vi "产生多组数值.vi"() -> (0 "牌3":dbl, 1 "牌4":dbl, 2 "牌2":dbl, 3 "牌1":dbl, 4 "牌4值":dbl, 5 "牌3值":dbl, 6 "牌2值":dbl, 7 "牌1值":dbl)   [LabVIEW 2014]
uses:
  <vilib>/Utility/file.llb/Write To Spreadsheet File (DBL).vi
panel:
  in  "数值":i32
  out "大小":i32[](array[numeric])
  out "添加的数组":dbl[][](array[numeric])
  out "布尔":bool
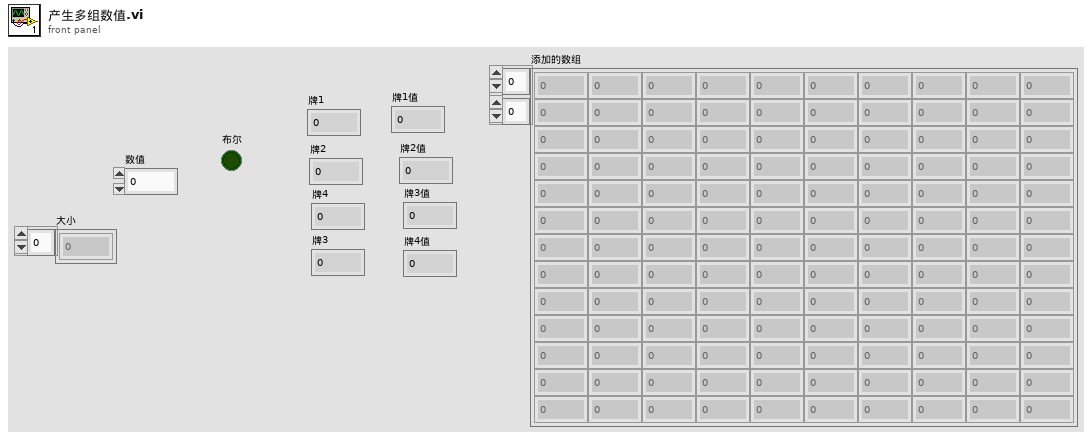
[diagram p1: front panel]
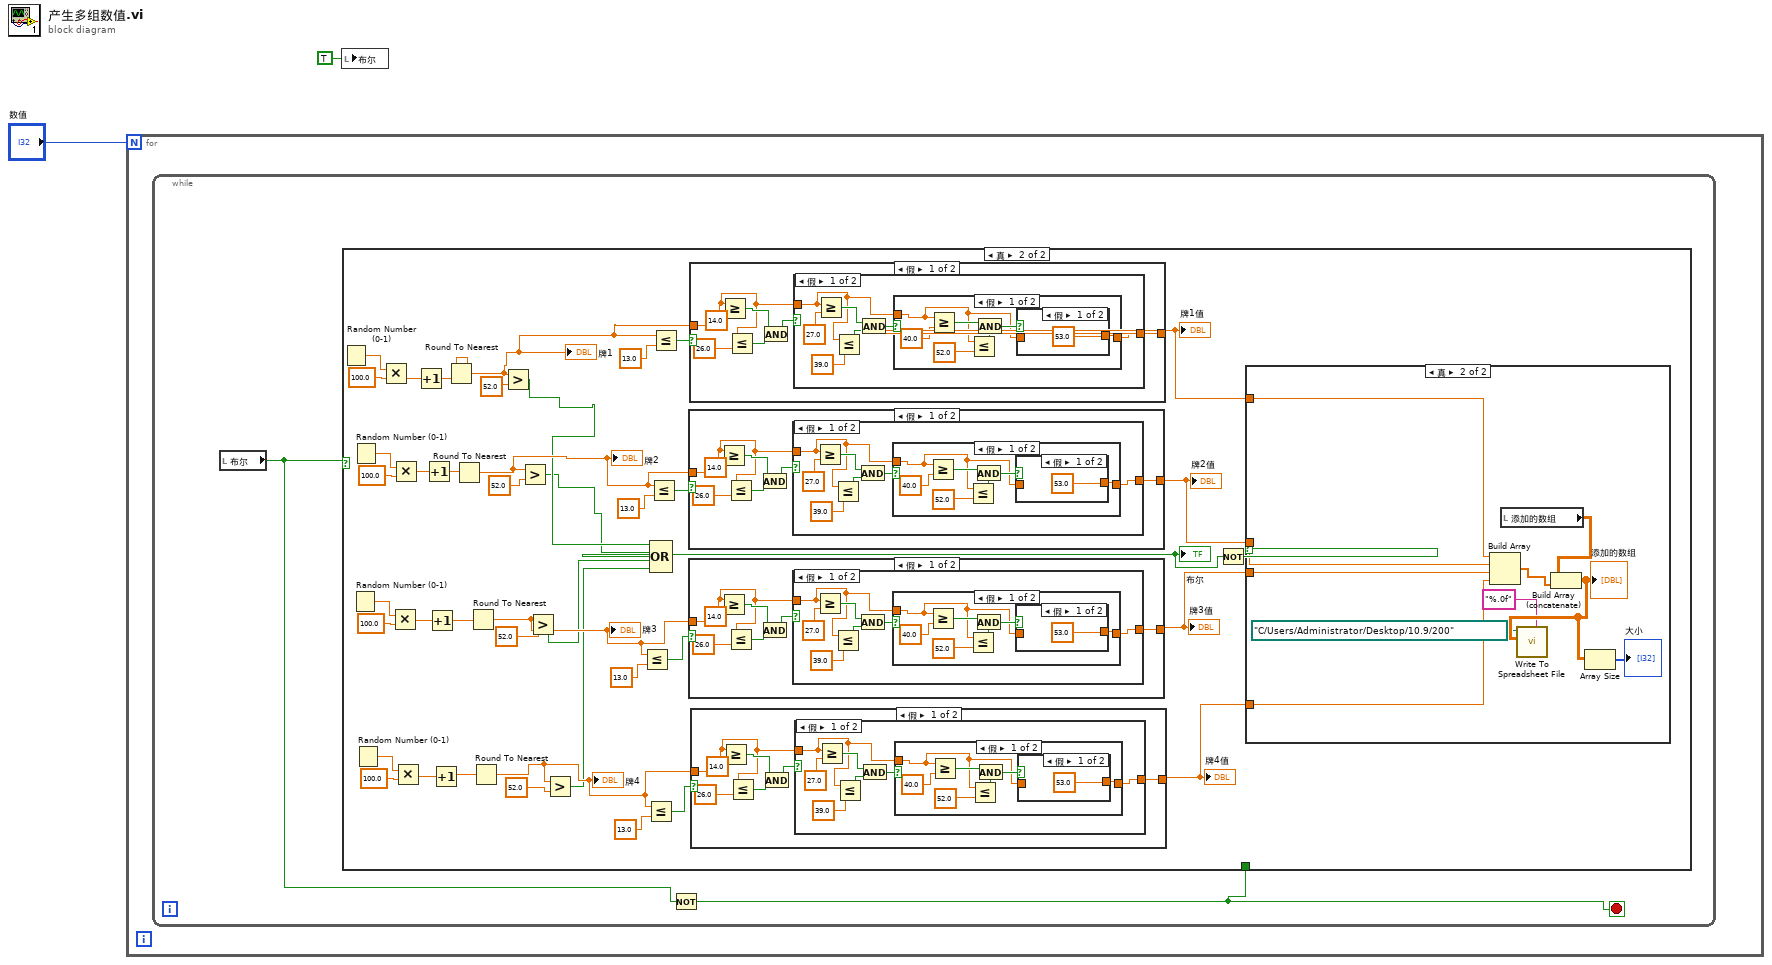
[diagram p0: block diagram]
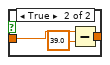
[diagram p4: hidden frame]
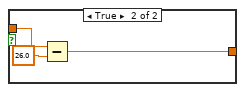
[diagram p5: hidden frame]
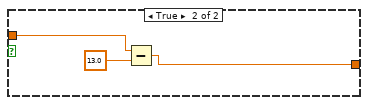
[diagram p6: hidden frame]
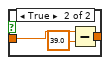
[diagram p8: hidden frame]
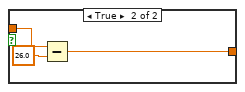
[diagram p9: hidden frame]
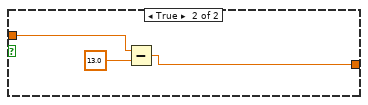
[diagram p10: hidden frame]
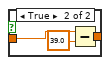
[diagram p12: hidden frame]
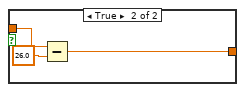
[diagram p13: hidden frame]
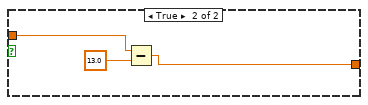
[diagram p14: hidden frame]
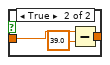
[diagram p16: hidden frame]
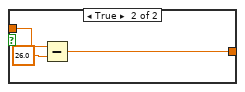
[diagram p17: hidden frame]
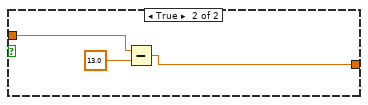
[diagram p18: hidden frame]
diagram:
  n1 = for {
    N: "数值" -> [_]
    n2 = while {
      stop <- w3 stop-if-true
      n3 = local read "布尔"() -> (w4:bool)
      n4 = Not(x=w4) -> (.not. x?=w3:bool)
      n5 = case shown="真" w4 {
        tunnel: w3 -> [_ _]
        frame False {
        }
        frame True {
          n6 = Random Number (0-1)() -> (number: 0 to 1=w39:dbl)
          n7 = Random Number (0-1)() -> (number: 0 to 1=w42:dbl)
          n8 = Random Number (0-1)() -> (number: 0 to 1=w46:dbl)
          n9 = Random Number (0-1)() -> (number: 0 to 1=w43:dbl)
          n10 = Multiply(x=w39, y=100.0) -> (x*y=w22:dbl)
          n11 = Multiply(x=w42, y=100.0) -> (x*y=w13:dbl)
          n12 = Multiply(x=w46, y=100.0) -> (x*y=w11:dbl)
          n13 = Multiply(x=w43, y=100.0) -> (x*y=w15:dbl)
          n14 = Increment(x=w22) -> (x+1=w21:dbl)
          n15 = Increment(x=w11) -> (x+1=w12:dbl)
          n16 = Increment(x=w13) -> (x+1=w14:dbl)
          n17 = Increment(x=w15) -> (x+1=w16:dbl)
          n18 = Round To Nearest(number=w21) -> (nearest integer value=w27:dbl)
          "牌1" <- w27
          n19 = Round To Nearest(number=w12) -> (nearest integer value=w28:dbl)
          "牌2" <- w28
          n20 = Round To Nearest(number=w14) -> (nearest integer value=w29:dbl)
          "牌3" <- w29
          n21 = Round To Nearest(number=w16) -> (nearest integer value=w30:dbl)
          "牌4" <- w30
          n22 = Greater?(x=w27, y=52.0) -> (0:w20:bool)
          n23 = Greater?(x=w28, y=52.0) -> (0:w19:bool)
          n24 = Greater?(x=w29, y=52.0) -> (0:w18:bool)
          n25 = Greater?(x=w30, y=52.0) -> (0:w17:bool)
          n26 = Less Or Equal?(x=w29, y=13.0) -> (x <= y?=w24:bool)
          n27 = Less Or Equal?(x=w30, y=13.0) -> (x <= y?=w23:bool)
          n28 = Less Or Equal?(x=w28, y=13.0) -> (x <= y?=w25:bool)
          n29 = Compound Arithmetic op=OR(w20, w19, w18, w17) -> (w6:bool)
          "布尔" <- w6
          n30 = Less Or Equal?(x=w27, y=13.0) -> (x <= y?=w26:bool)
          n31 = case shown="假" w25 {
            tunnel: [w121 w152] -> w9
            tunnel: w28 -> [w122 w152]
            frame False {
              n32 = Greater Or Equal?(x=w122, y=14.0) -> (x >= y?=w124:bool)
              n33 = Less Or Equal?(x=w122, y=26.0) -> (x <= y?=w125:bool)
              n34 = And(x=w124, y=w125) -> (x .and. y?=w123:bool)
              n35 = case shown="假" w123 {
                tunnel: w122 -> [w129 w150]
                tunnel: [w128 w149] -> w121
                frame False {
                  n36 = Greater Or Equal?(x=w129, y=27.0) -> (x >= y?=w132:bool)
                  n37 = Less Or Equal?(x=w129, y=39.0) -> (x <= y?=w131:bool)
                  n38 = And(x=w132, y=w131) -> (x .and. y?=w130:bool)
                  n39 = case shown="假" w130 {
                    tunnel: w129 -> [w137 w148]
                    tunnel: [w136 w146] -> w128
                    frame False {
                      n40 = Greater Or Equal?(x=w137, y=40.0) -> (x >= y?=w139:bool)
                      n41 = Less Or Equal?(x=w137, y=52.0) -> (x <= y?=w135:bool)
                      n42 = And(x=w139, y=w135) -> (x .and. y?=w138:bool)
                      n43 = case shown="假" w138 {
                        tunnel: w137 -> [_ w144]
                        tunnel: [53.0 ("y") w143] -> w136
                        frame False {
                        }
                        frame True {
                          n44 = Subtract(x=w144, y=39.0) -> (x-y=w143:dbl)
                        }
                      }
                    }
                    frame True {
                      n45 = Subtract(x=w148, y=26.0) -> (x-y=w146:dbl)
                    }
                  }
                }
                frame True {
                  n46 = Subtract(x=w150, y=13.0) -> (x-y=w149:dbl)
                }
              }
            }
            frame True {
            }
          }
          "牌2值" <- w9
          n47 = case shown="假" w24 {
            tunnel: [w89 w120] -> w8
            tunnel: w29 -> [w90 w120]
            frame False {
              n48 = Greater Or Equal?(x=w90, y=14.0) -> (x >= y?=w92:bool)
              n49 = Less Or Equal?(x=w90, y=26.0) -> (x <= y?=w93:bool)
              n50 = And(x=w92, y=w93) -> (x .and. y?=w91:bool)
              n51 = case shown="假" w91 {
                tunnel: w90 -> [w97 w118]
                tunnel: [w96 w117] -> w89
                frame False {
                  n52 = Greater Or Equal?(x=w97, y=27.0) -> (x >= y?=w100:bool)
                  n53 = Less Or Equal?(x=w97, y=39.0) -> (x <= y?=w99:bool)
                  n54 = And(x=w100, y=w99) -> (x .and. y?=w98:bool)
                  n55 = case shown="假" w98 {
                    tunnel: w97 -> [w105 w116]
                    tunnel: [w104 w114] -> w96
                    frame False {
                      n56 = Greater Or Equal?(x=w105, y=40.0) -> (x >= y?=w107:bool)
                      n57 = Less Or Equal?(x=w105, y=52.0) -> (x <= y?=w103:bool)
                      n58 = And(x=w107, y=w103) -> (x .and. y?=w106:bool)
                      n59 = case shown="假" w106 {
                        tunnel: w105 -> [_ w112]
                        tunnel: [53.0 ("y") w111] -> w104
                        frame False {
                        }
                        frame True {
                          n60 = Subtract(x=w112, y=39.0) -> (x-y=w111:dbl)
                        }
                      }
                    }
                    frame True {
                      n61 = Subtract(x=w116, y=26.0) -> (x-y=w114:dbl)
                    }
                  }
                }
                frame True {
                  n62 = Subtract(x=w118, y=13.0) -> (x-y=w117:dbl)
                }
              }
            }
            frame True {
            }
          }
          "牌3值" <- w8
          n63 = case shown="假" w26 {
            tunnel: [w153 w184] -> w10
            tunnel: w27 -> [w154 w184]
            frame False {
              n64 = Greater Or Equal?(x=w154, y=14.0) -> (x >= y?=w156:bool)
              n65 = Less Or Equal?(x=w154, y=26.0) -> (x <= y?=w157:bool)
              n66 = And(x=w156, y=w157) -> (x .and. y?=w155:bool)
              n67 = case shown="假" w155 {
                tunnel: w154 -> [w161 w182]
                tunnel: [w160 w181] -> w153
                frame False {
                  n68 = Greater Or Equal?(x=w161, y=27.0) -> (x >= y?=w164:bool)
                  n69 = Less Or Equal?(x=w161, y=39.0) -> (x <= y?=w163:bool)
                  n70 = And(x=w164, y=w163) -> (x .and. y?=w162:bool)
                  n71 = case shown="假" w162 {
                    tunnel: w161 -> [w169 w180]
                    tunnel: [w168 w178] -> w160
                    frame False {
                      n72 = Greater Or Equal?(x=w169, y=40.0) -> (x >= y?=w171:bool)
                      n73 = Less Or Equal?(x=w169, y=52.0) -> (x <= y?=w167:bool)
                      n74 = And(x=w171, y=w167) -> (x .and. y?=w170:bool)
                      n75 = case shown="假" w170 {
                        tunnel: w169 -> [_ w176]
                        tunnel: [53.0 ("y") w175] -> w168
                        frame False {
                        }
                        frame True {
                          n76 = Subtract(x=w176, y=39.0) -> (x-y=w175:dbl)
                        }
                      }
                    }
                    frame True {
                      n77 = Subtract(x=w180, y=26.0) -> (x-y=w178:dbl)
                    }
                  }
                }
                frame True {
                  n78 = Subtract(x=w182, y=13.0) -> (x-y=w181:dbl)
                }
              }
            }
            frame True {
            }
          }
          "牌1值" <- w10
          n79 = case shown="假" w23 {
            tunnel: [w57 w88] -> w7
            tunnel: w30 -> [w58 w88]
            frame False {
              n80 = Greater Or Equal?(x=w58, y=14.0) -> (x >= y?=w60:bool)
              n81 = Less Or Equal?(x=w58, y=26.0) -> (x <= y?=w61:bool)
              n82 = And(x=w60, y=w61) -> (x .and. y?=w59:bool)
              n83 = case shown="假" w59 {
                tunnel: w58 -> [w65 w86]
                tunnel: [w64 w85] -> w57
                frame False {
                  n84 = Greater Or Equal?(x=w65, y=27.0) -> (x >= y?=w68:bool)
                  n85 = Less Or Equal?(x=w65, y=39.0) -> (x <= y?=w67:bool)
                  n86 = And(x=w68, y=w67) -> (x .and. y?=w66:bool)
                  n87 = case shown="假" w66 {
                    tunnel: w65 -> [w73 w84]
                    tunnel: [w72 w82] -> w64
                    frame False {
                      n88 = Greater Or Equal?(x=w73, y=40.0) -> (x >= y?=w75:bool)
                      n89 = Less Or Equal?(x=w73, y=52.0) -> (x <= y?=w71:bool)
                      n90 = And(x=w75, y=w71) -> (x .and. y?=w74:bool)
                      n91 = case shown="假" w74 {
                        tunnel: w73 -> [_ w80]
                        tunnel: [53.0 ("y") w79] -> w72
                        frame False {
                        }
                        frame True {
                          n92 = Subtract(x=w80, y=39.0) -> (x-y=w79:dbl)
                        }
                      }
                    }
                    frame True {
                      n93 = Subtract(x=w84, y=26.0) -> (x-y=w82:dbl)
                    }
                  }
                }
                frame True {
                  n94 = Subtract(x=w86, y=13.0) -> (x-y=w85:dbl)
                }
              }
            }
            frame True {
            }
          }
          "牌4值" <- w7
          n95 = Not(x=w6) -> (.not. x?=w5:bool)
          n96 = case shown="真" w5 {
            tunnel: w10 -> [_ w56]
            tunnel: w9 -> [_ w55]
            tunnel: w8 -> [_ w54]
            tunnel: w7 -> [_ w53]
            frame False {
            }
            frame True {
              n97 = Build Array(w56, w55, w54, w53) -> (w52:dbl[])
              n98 = local read "添加的数组"() -> (w51:dbl[][])
              n99 = Build Array (concatenate)(w51, w52) -> (w49:dbl[][])
              "添加的数组" <- w49
              n100 = call-poly <vilib>:"Write To Spreadsheet File.vi"("format (%.3f)"="%.0f", "2D data"=w49, "file path (dialog if empty)"=path "C:/Users/Administrator/Desktop/10.9/200") -> ()  [unwired: 5 in, 1 out]
              n101 = Array Size(array=w49) -> (size(s)=→"大小":i32[])
            }
          }
        }
      }
    }
  }
  n102 = local write "布尔"(TRUE ("布尔")) -> ()
